vi "(Var) Chamber.vi"() -> ()   [LabVIEW 2017]
panel:
  out "Run ?":bool
  out "Chamber Temp":dbl format="%.2f ∩"
  in  "Target Temp":u16 format="%d ∩"
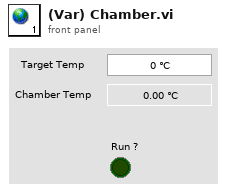
[diagram p1: front panel]
diagram:
